vi "SousVi.vi"(1 "Numérique":i32) -> (0 "Tableau":dbl[](array[numeric]))   [LabVIEW 2018]
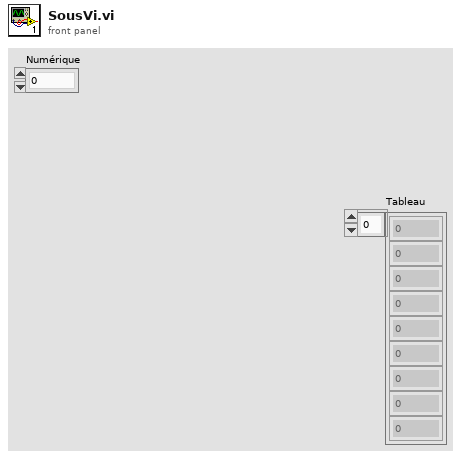
[diagram p1: front panel]
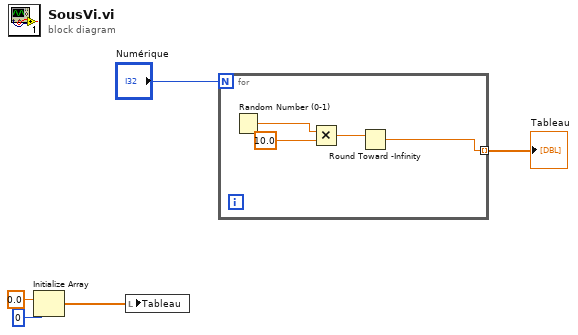
[diagram p0: block diagram]
diagram:
  n1 = Initialize Array(0.0 ("élément"), 0 ("taille de la dimension")) -> (w3:dbl[])
  n2 = local write "Tableau"(w3) -> ()
  n3 = for {
    N: "Numérique" -> [_]
    tunnel: [w6] -> w1 mode=indexing
    n4 = Random Number (0-1)() -> (number: 0 to 1=w8:dbl)
    n5 = Multiply(x=w8, y=10.0) -> (x*y=w7:dbl)
    n6 = Round Toward -Infinity(1:w7) -> (0:w6:dbl)
  }
  "Tableau" <- w1
